vi "Read XML_Parse Dot Net Error.vi"(11 "error in (no error)":errorcluster) -> (3 "error out":errorcluster)   [LabVIEW 2020]
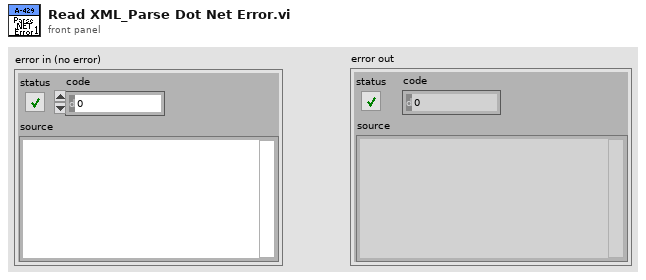
[diagram p1: front panel]
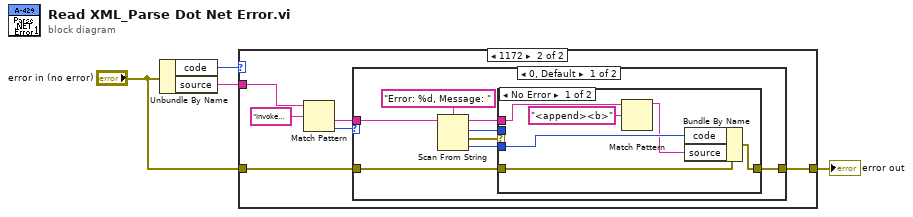
[diagram p0: block diagram]
diagram:
  n1 = Unbundle By Name("error in (no error)") -> ("code"=w4:i32, "source"=w3:string)
  n2 = case shown="1172" w4 {
    tunnel: w3 -> [_ w10]
    tunnel: "error in (no error)" -> [w5 w7]
    tunnel: [w5 w6] -> w1
    frame 0, Default {
    }
    frame 1172 {
      n3 = Match Pattern(string=w10, regular expression="Invoke Node System.Reflection.TargetInvocationException: Exception has been thrown by the target of an invocation.\n\tInner Exception: System.ApplicationException: \n\n" ("name")) -> (after substring=w8:string, offset past match=w9:i32)  [unwired: 1 in, 2 out]
      n4 = case shown="0, Default" w9 {
        tunnel: w8 -> [w19 _]
        tunnel: w7 -> [w16 w27]
        tunnel: [w15 w27] -> w6
        frame 0, Default {
          n5 = Scan From String(format string="Error: %d, Message: ", input string=w19) -> (remaining string=w12:string, offset past scan=w13:u32, error out=w17:errorcluster, output 1=w14:i32)  [unwired: 3 in]
          n6 = case shown="No Error" w17 {
            tunnel: w16 -> [w25 w26]
            tunnel: [w24 w26] -> w15
            tunnel: w14 -> [w23 _]
            tunnel: w13 -> [_ _]
            tunnel: w12 -> [w22 _]
            frame No Error {
              n7 = Match Pattern(string=w22, regular expression="<append><b>") -> (before substring=w20:string)  [unwired: 1 in, 3 out]
              n8 = Bundle By Name(cluster=w25, "code"=w23, "source"=w20) -> (w24:errorcluster)
            }
            frame Error {
            }
          }
        }
        frame -1 {
        }
      }
    }
  }
  "error out" <- w1
